vi "FMTone-Initialize.vi"(0 "FM":T1, 7 "Sampling rate (Hz)":dbl, 9 "Npts":i32, 11 "error in (no error)":errorcluster) -> (15 "error out":errorcluster)   [LabVIEW 2020]
uses:
  XControls/Waveform XControls/FM Tone/Data.ctl
  XControls/Waveform XControls/FM Tone/FM Tone.xctl
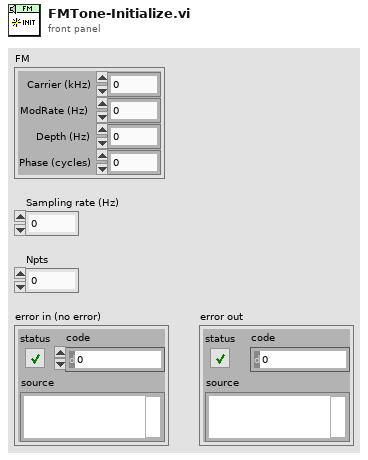
[diagram p1: front panel]
types:
  T1 = typedef "FM Tone.xctl/Data.ctl" = cluster{"Carrier (kHz)":dbl, "ModRate (Hz)":dbl, "Depth (Hz)":dbl, "Phase (cycles)":dbl}
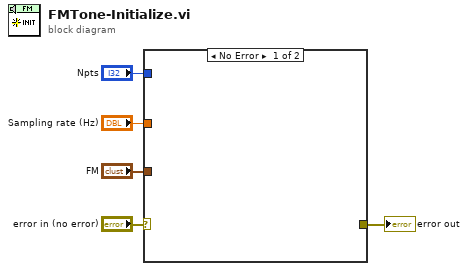
[diagram p0: block diagram]
diagram:
  n1 = case shown="No Error" "error in (no error)" {
    selector: "error in (no error)" -> [_ w6]
    tunnel: [_ w6] -> w2
    tunnel: "Sampling rate (Hz)" -> [_ _]
    tunnel: "Npts" -> [_ _]
    tunnel: "FM" -> [_ _]
    frame No Error {
    }
    frame Error {
    }
  }
  "error out" <- w2
